vi "Send SetHistogramParameter.vi"(6 "tacq":i32, 7 "Message Priority (Normal)":T1=enum."Normal", 8 "error in (no error)":errorcluster, 9 "Value":i32, 10 "Parameter":enum16{"HistoLen", "HistoOffset", "Binning"}(ring)=enum."Binning", 11 "Message Enqueuer":refnum<class "Message Enqueuer.lvclass">) -> (0 "error out":errorcluster, 3 "Message Enqueuer out":refnum<class "Message Enqueuer.lvclass">)   [LabVIEW 2023, in "Multiharp.lvlib" / "SetHistogramParameter Msg.lvclass"]
doc: "This VI sends the message to an actor."
uses:
  SetHistogramParameter Msg.lvclass
  <vilib>/ActorFramework/Message Enqueuer/Message Enqueuer.lvclass
  <vilib>/ActorFramework/Message Enqueuer/Message Priority.ctl
  SetHistogramParameter Msg.lvclass/SetHistogramParameter Msg.ctl
  <vilib>/ActorFramework/Message Enqueuer/Message Enqueuer.lvclass/Message Enqueuer.ctl
  <vilib>/ActorFramework/Message Priority Queue/Priority Enqueue.vi
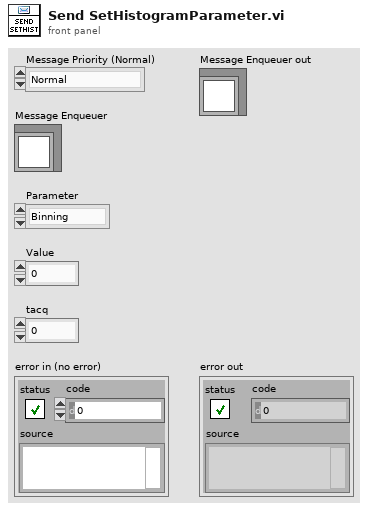
[diagram p1: front panel]
types:
  T1 = typedef "Actor Framework.lvlib/Message Enqueuer.lvclass/Message Priority.ctl" = enum16{"Low", "Normal", "High"}
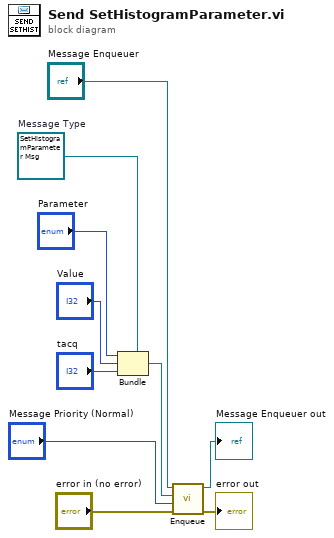
[diagram p0: block diagram]
diagram:
  w4 = refnum<class "SetHistogramParameter Msg.lvclass"> refnum  # Message Type
  n1 = Bundle(cluster=w4, "Parameter", "Value", "tacq") -> (w5:refnum<class "SetHistogramParameter Msg.lvclass">)
  n2 = call <vilib>:"Enqueue.vi"("error in (no error)"="error in (no error)", "Message Priority (Normal)"="Message Priority (Normal)", "Message"=w5, "Message Enqueuer in"="Message Enqueuer") -> ("error out"=→"error out":errorcluster, "Message Enqueuer out"=→"Message Enqueuer out":refnum<class "Message Enqueuer.lvclass">)  [unwired: 6 in]
